vi "emi_Is Dev enviroment.vi"(9 "error in (no error)":errorcluster) -> (8 "Dev System?":bool, 10 "error out":errorcluster)   [LabVIEW 2011]
doc: "Returns true if the VI is running in the development enviroment.\n\nDoes not include error terminals to maximise performance.\n\nSubroutine"
panel:
  # "conditional disable klart raskes.\nFB er ikke langt etter"
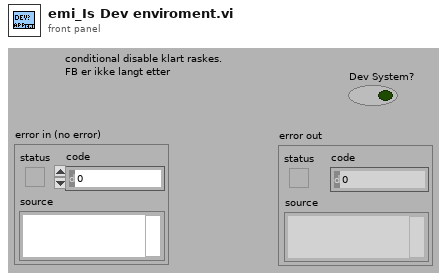
[diagram p1: front panel]
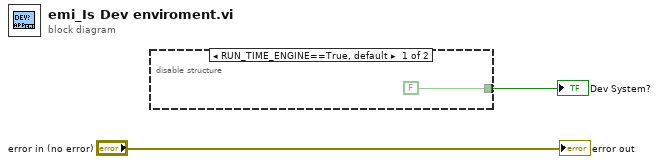
[diagram p0: block diagram]
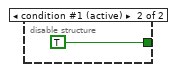
[diagram p2: hidden frame]
diagram:
  n1 = disable-structure shown="RUN_TIME_ENGINE==True, default" {
    disable-tunnel: [FALSE TRUE ("Boolean")] -> w2
    frame condition #0 {
    }
    frame condition #1 (active) {
    }
  }
  "Dev System?" <- w2
  "error out" <- "error in (no error)"
